vi "ASDA-A2_Connect.vi"(8 "error in":errorcluster, 10 "Connection Data":T1={"COM Port"="", "Baud Rate"=115200, "Unit ID"=1}, 11 "Buffer Data In":T2) -> (0 "error out":errorcluster, 3 "Buffer Data Out":T2)   [LabVIEW 2016]
uses:
  Data Def/ASDA-A2_Buffer Data.ctl
  Data Def/ASDA-A2_Connection Data.ctl
  <vilib>/Modbus/master/Create Master Instance (Serial).vi
  <vilib>/Modbus/master/Modbus Master.lvclass
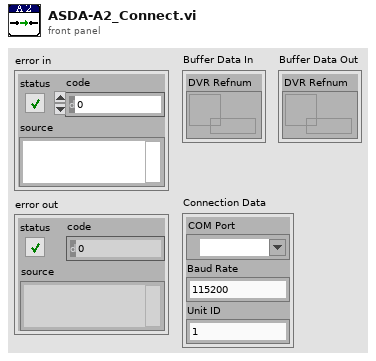
[diagram p1: front panel]
types:
  T1 = typedef "ASDA-A2_Connection Data.ctl" = cluster{"COM Port":refnum<visa-resource-name>, "Baud Rate":u32, "Unit ID":u8}
  T2 = typedef "ASDA-A2_Buffer Data.ctl" = cluster{"DVR Refnum":refnum<data-value>}
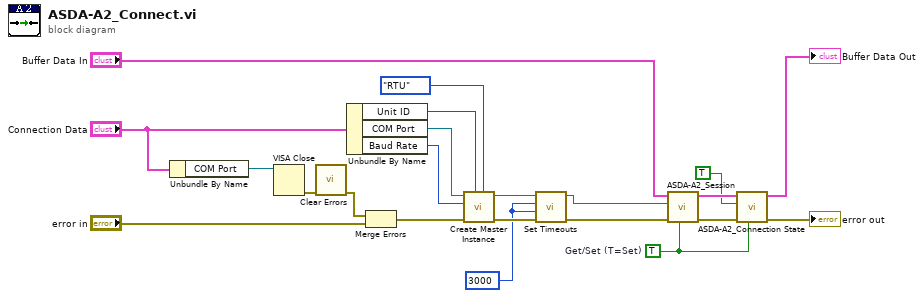
[diagram p0: block diagram]
diagram:
  w5 = 3000 ("Write Timeout")
  w9 = TRUE  # Get/Set (T=Set)
  n1 = Unbundle By Name("Connection Data") -> ("COM Port"=w15:refnum<visa-resource-name>)
  n2 = VISA Close(VISA resource name=w15) -> (error out=w16:errorcluster)  [unwired: 1 in]
  n3 = call <vilib>:"Clear Errors.vi"("error in (no error)"=w16) -> ("error out"=w13:errorcluster)  [unwired: 5 in, 1 out]
  n4 = Unbundle By Name("Connection Data") -> ("Unit ID"=w22:u8, "COM Port"=w20:refnum<visa-resource-name>, "Baud Rate"=w19:u32)
  n5 = Merge Errors(w13, "error in") -> (w14:errorcluster)
  n6 = call-poly <vilib>:"Create Master Instance.vi"("serial type"=enum16{"RTU", "ASCII"}."RTU", "unit ID"=w22, "error in (no error)"=w14, "baud rate (9600)"=w19, "VISA resource name"=w20) -> ("error out"=w7:errorcluster, "serial master instance"=w6:refnum<class "Modbus Master.lvclass">)  [unwired: 5 in]
  n7 = call <vilib>:"Set Timeouts.vi"("error in (no error)"=w7, "write operation timeout (ms)"=w5, "read operation timeout (ms)"=w5, "Modbus master in"=w6) -> ("error out"=w4:errorcluster, "Modbus master out"=w3:refnum<class "Modbus Master.lvclass">)  [unwired: 6 in]
  n8 = call "ASDA-A2_Session.vi"("Get/Set (T=Set)"=w9, "error in"=w4, "Session In"=w3, "Buffer Data In"="Buffer Data In") -> ("error out"=w11:errorcluster, "Buffer Data Out"=w10:T2)  [unwired: 5 in, 1 out]
  n9 = call "ASDA-A2_Connection State.vi"("Get/Set (T=Set)"=w9, "error in"=w11, "State In"=TRUE, "Buffer Data In"=w10) -> ("error out"=→"error out":errorcluster, "Buffer Data Out"=→"Buffer Data Out":T2)  [unwired: 5 in, 1 out]
